vi "Hide.vi"(8 "error in":errorcluster, 11 "Flex Subpanel in":refnum<class "Flex UI Subpanel.lvclass">) -> (0 "error out":errorcluster, 3 "Flex Subpanel out":refnum<class "Flex UI Subpanel.lvclass">)   [LabVIEW 2016, in "Flex UI Subpanel.lvclass"]
doc: "Hides the UI."
uses:
  Flex UI Subpanel.lvclass
  Flex UI Subpanel.lvclass/Flex UI Subpanel.ctl
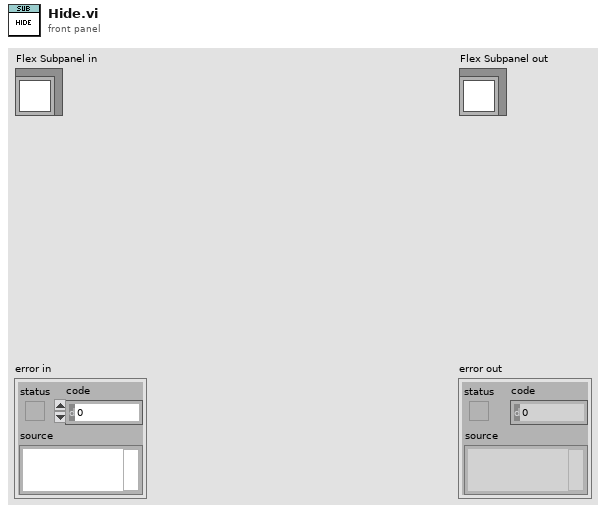
[diagram p1: front panel]
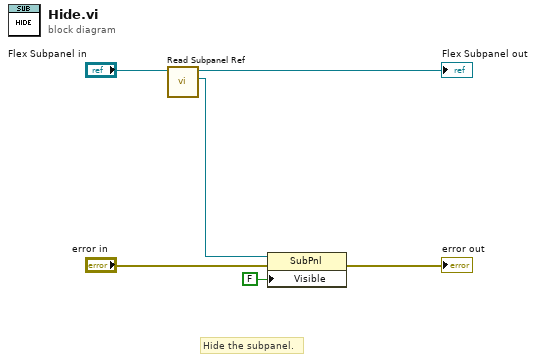
[diagram p0: block diagram]
diagram:
  # "Hide the subpanel."
  n1 = call "Read Subpanel Ref.vi"("Flex Subpanel in"="Flex Subpanel in") -> ("Subpanel Ref"=w3:refnum<vi>, "Flex Subpanel out"=→"Flex Subpanel out":refnum<class "Flex UI Subpanel.lvclass">)  [unwired: 9 in]
  n2 = property class="SubPnl"(reference=w3, error in="error in", "Visible"=FALSE) -> (error out=→"error out":errorcluster)  [unwired: 1 out]
